vi "Acquire Module Semaphore.vi"(8 "error in":errorcluster) -> (0 "error out":errorcluster)   [LabVIEW 2024, in "Chart.lvlib"]
doc: "Acquire the module semaphore.\n_____\nCreated using DQMH Event Scripter 6.1.0.128."
uses:
  Chart.lvlib
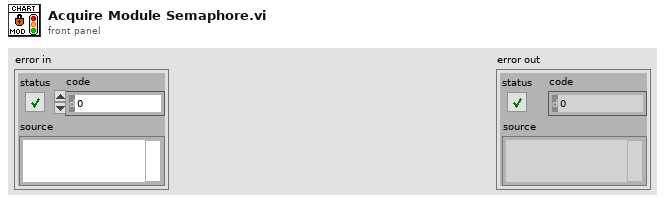
[diagram p1: front panel]
types:
  T1 = typedef "Semaphore RefNum" = refnum<k1>
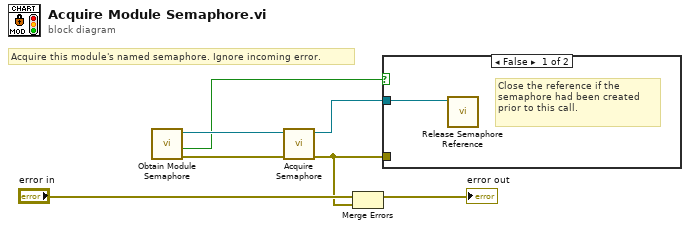
[diagram p0: block diagram]
diagram:
  # "Acquire this module's named semaphore. Ignore incoming error."
  n1 = call "Obtain Module Semaphore.vi"() -> ("error out"=w7:errorcluster, "created new"=w3:bool, "semaphore"=w6:T1)  [unwired: 9 in]
  n2 = call <vilib>:"Acquire Semaphore.vi"("error in (no error)"=w7, "semaphore"=w6) -> ("error out"=w1:errorcluster, "semaphore out"=w2:T1)  [unwired: 3 in, 1 out]
  n3 = Merge Errors("error in", w1) -> (→"error out":errorcluster)
  n4 = case shown="False" w3 {
    tunnel: w2 -> [w8 _]
    tunnel: w1 -> [_ _]
    frame False {
      # "Close the reference if the semaphore had been created prior to this call."
      n5 = call <vilib>:"Release Semaphore Reference.vi"("semaphore"=w8) -> ()  [unwired: 9 in, 2 out]
    }
    frame True {
    }
  }
